vi "Test Monitoring.vi"(8 "error in":errorcluster, 9 "Duration(sec)":u16=1000, 10 "Socket":string, 11 "SequenceContext":refnum<k7>) -> (0 "Error Out":errorcluster)   [LabVIEW 2021, in "Display.lvlib"]
doc: "This VI loops until either the Stop button is pressed or the calling TestStand sequence is terminated. The Termination Monitor VI allows this VI to query the TestStand execution for its current status."
uses:
  Display.lvlib
panel:
  out "Messages":string="0  00:01:15"
  in  "Stop Button":bool
  out "Test Steps":T1
  out "Elapsed Time":string="0  00:01:15"
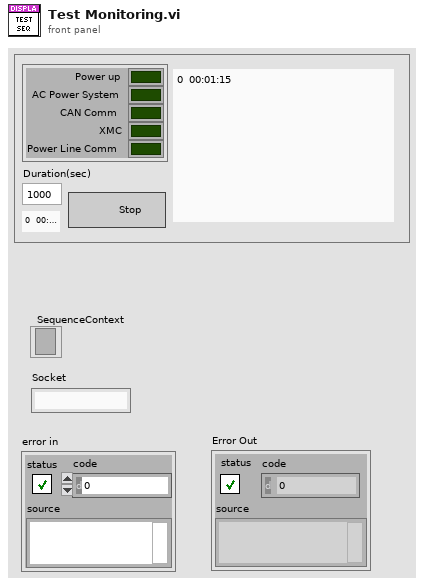
[diagram p1: front panel]
types:
  T1 = cluster{"Power up":bool, "AC Power System":bool, "CAN Comm":bool, "XMC":bool, "Power Line Comm":bool}
  T2 = typedef "TestStand - Status Monitor.ctl" = cluster{"Sequence Context":refnum<k7>, "Execution":refnum<k7>, "Termination Monitor":refnum<k7>}
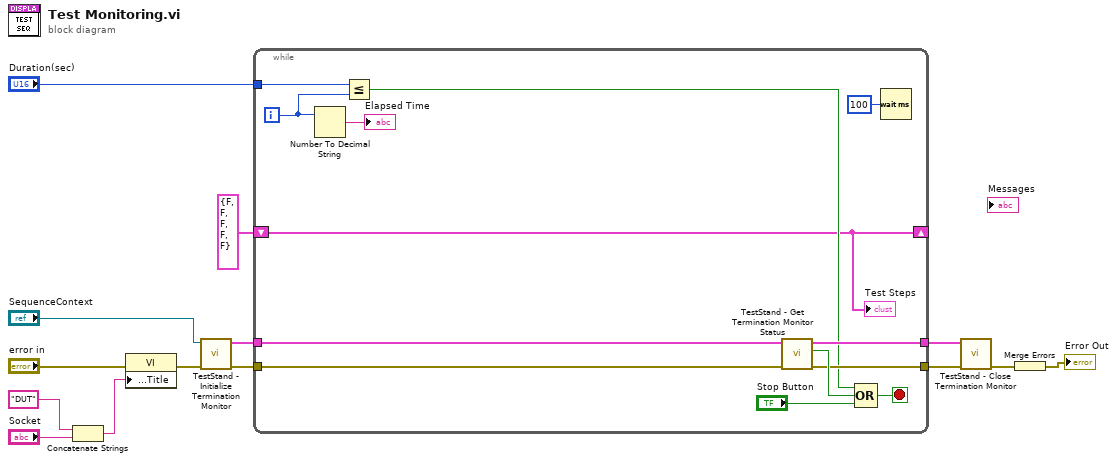
[diagram p0: block diagram]
diagram:
  n1 = Concatenate Strings("DUT" ("string"), "Socket") -> (w5:string)
  n2 = property class="VI"(error in="error in", "Front Panel.Title"=w5) -> (error out=w2:errorcluster)  [unwired: 1 in, 1 out]
  n3 = call <vilib>:"TestStand - Initialize Termination Monitor.vi"("error in (no error)"=w2, "Sequence Context In"="SequenceContext") -> ("error out"=w10:errorcluster, "Status Monitor Out"=w9:T2)  [unwired: 8 in]
  n4 = while {
    tunnel: w9 -> [w27]
    tunnel: [w26] -> w6
    tunnel: w10 -> [w24]
    tunnel: [w22] -> w7
    tunnel: "Duration(sec)" -> [w20]
    shift-right: [w16] -> _
    shift-left: T1 {"Power up"=FALSE, "AC Power System"=FALSE, "CAN Comm"=FALSE, "XMC"=FALSE, "Power Line Comm"=FALSE} ("Test Steps") -> [w16]
    i -> [w15]
    stop <- w25 stop-if-true
    n5 = Number To Decimal String(number=w15) -> (decimal integer string=→"Elapsed Time":string)  [unwired: 1 in]
    n6 = Less Or Equal?(x=w20, y=w15) -> (x <= y?=w19:bool)
    n7 = call <vilib>:"TestStand - Get Termination Monitor Status.vi"("error in (no error)"=w24, "Status Monitor In"=w27) -> ("error out"=w22:errorcluster, "Terminating or Aborting"=w23:bool, "Status Monitor Out"=w26:T2)  [unwired: 7 in]
    n8 = Compound Arithmetic op=OR(w19, w23, "Stop Button") -> (w25:bool)
    n9 = Wait (ms)(milliseconds to wait=u32 100) -> ()  [unwired: 1 out]
    "Test Steps" <- w16
  }
  n10 = call <vilib>:"TestStand - Close Termination Monitor.vi"("error in (no error)"=w7, "Status Monitor In"=w6) -> ("error out"=w8:errorcluster)  [unwired: 9 in]
  n11 = Merge Errors(w8) -> (→"Error Out":errorcluster)
